vi "Set Inputs.vi"(6 "uService ID (optional)":string, 7 "Highlander?":bool, 8 "error in (no error)":errorcluster, 9 "GUI?":bool, 10 "uService Class Name":string, 11 "Launch uService Msg in":refnum<class "Launch uService Msg.lvclass">) -> (0 "error out":errorcluster, 3 "Launch uService Msg out":refnum<class "Launch uService Msg.lvclass">)   [LabVIEW 2026, in "TALOS.lvlib" / "Guardian.lvlib" / "Launch uService Msg.lvclass"]
uses:
  Launch uService Msg.lvclass
  Launch uService Msg.lvclass/Launch uService Msg.ctl
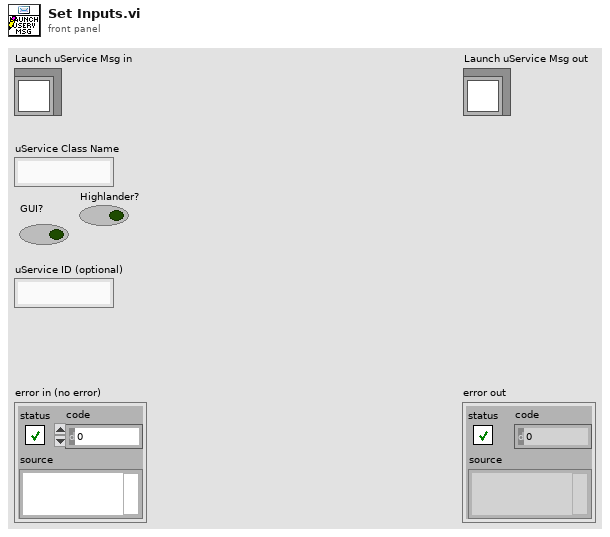
[diagram p1: front panel]
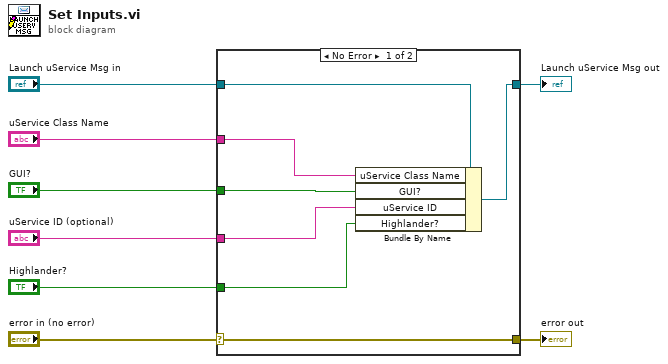
[diagram p0: block diagram]
diagram:
  n1 = case shown="No Error" "error in (no error)" {
    selector: "error in (no error)" -> [w15 w16]
    tunnel: [w15 w16] -> w7
    tunnel: [w13 w17] -> w5
    tunnel: "Launch uService Msg in" -> [w14 w17]
    tunnel: "uService Class Name" -> [w12 _]
    tunnel: "GUI?" -> [w11 _]
    tunnel: "uService ID (optional)" -> [w10 _]
    tunnel: "Highlander?" -> [w9 _]
    frame No Error {
      n2 = Bundle By Name(cluster=w14, "uService Class Name"=w12, "GUI?"=w11, "uService ID"=w10, "Highlander?"=w9) -> (w13:refnum<class "Launch uService Msg.lvclass">)
    }
    frame Error {
    }
  }
  "error out" <- w7
  "Launch uService Msg out" <- w5
